vi "tm_getrange_a.vi"(8 "error in (no error)":errorcluster, 10 "Parameter":u32(ring)=4215968 items=["SENSOR MODE"=4212128, "CCD MODE"=4212384, "READOUT MODE"=4211872, "ACTIVE VIEW INDEX"=4343136, "BITS PER CHANNEL"=4342976, "IMAGE PIXEL TYPE"=4343296, "BINNING"=4215968, "EXPOSURE TIME"=2049184, "CONTRAST GAIN"=3163312, "CONTRAST OFFSET"=3163328, "LIGHT MODE"=2114720, "SENSITIVITY"=2114992, "PHOTON IMAGING MODE"=2115200, "HIGH DYNAMIC RANGE MODE"=3163360, "WHITE BALANCE"=3163568, "TEMPERATURE"=2115232, "TEMPERATURE TARGET"=2115264, "SENSOR COOLER FAN"=2115296, "LINEBUNDLE HEIGHT"=4212192, "MECHANICAL SHUTTER"=2115488, "BACK FOCUS POSITION"=8422304, "TRIGGER CONNECTOR"=1066432, "TRIGGER SOURCE"=1066144, "OUTPUT TRIGGER SOURCE"=1852576, "TRIGGER GLOBAL EXPOSURE"=2049680, "FIRST TRIGGER BEHAVIOR"=2049696, "CHANNEL SYNC"=1852352, "READOUT DIRECTION"=4211904, "PRE HSYNC COUNT"=1852704, "INTERNAL LINE SPEED"=4191408, "INTERNAL LINE INVERVAL"=4191424], 11 "Handle in":u32) -> (0 "error out":errorcluster, 1 "default":dbl, 2 "Range":cluster{"min":dbl, "max":dbl, "step":dbl}, 3 "Handle out":u32, 4 "Value Names":cluster{"Name":string, "Value":dbl}[](array[cluster]), 5 "Writable":bool, 6 "Text Values":bool)   [LabVIEW 2012]
uses:
  tmcamcon.dll
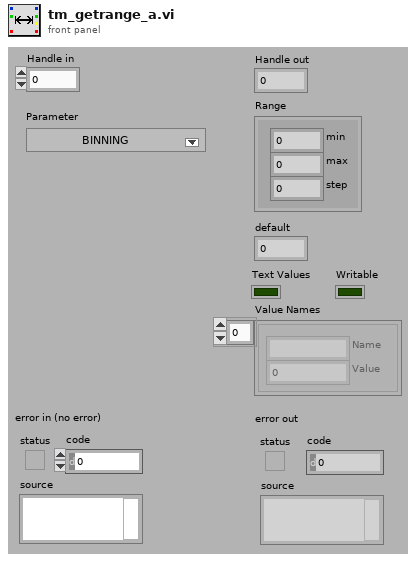
[diagram p1: front panel]
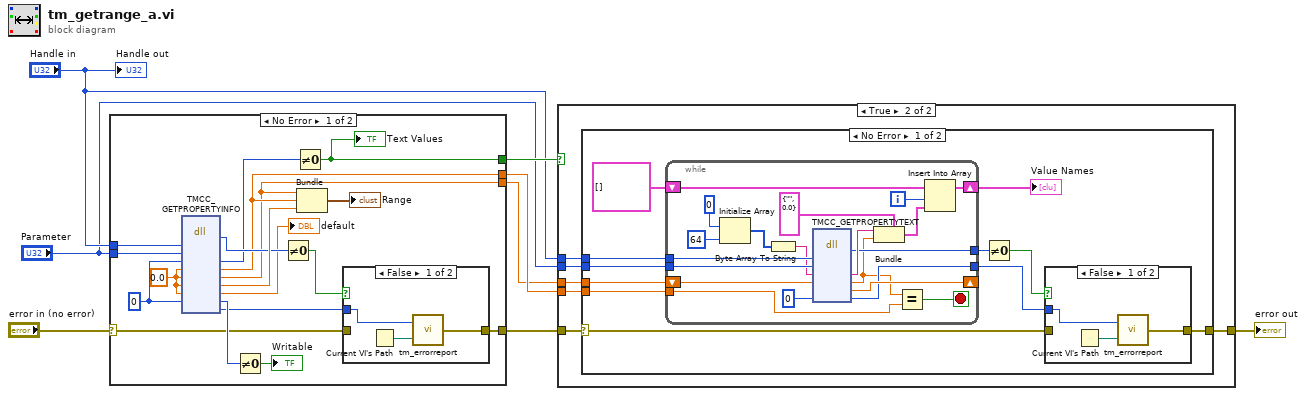
[diagram p0: block diagram]
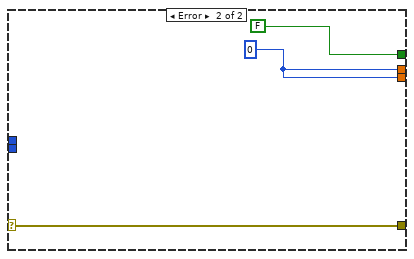
[diagram p6: hidden frame]
diagram:
  n1 = case shown="No Error" "error in (no error)" {
    selector: "error in (no error)" -> [w12 w33]
    tunnel: [w9 w33] -> w6
    tunnel: "Parameter" -> [w26 _]
    tunnel: "Handle in" -> [w20 _]
    tunnel: [w18 w31] -> w4
    tunnel: [w17 w31] -> w3
    tunnel: [w19 FALSE] -> w7
    frame No Error {
      w25 = 0.0
      w13 = u32 0
      n2 = dll-call lib="tmcamcon.dll" fn="TMCC_GETPROPERTYINFO"("HDCAM"=w20, "propertyid"=w26, "text"=w13, "max"=w25, "min"=w25, "step"=w25, "default"=w25, "writable"=w13) -> (w22:u32, "text"=w21:u32, "max"=w18:dbl, "min"=w17:dbl, "step"=w23:dbl, "default"=→"default":dbl, "writable"=w14:u32, "Erval"=w11:i32)  [unwired: 6 in, 2 out]
      n3 = Not Equal To 0?(x=w14) -> (x != 0?=→"Writable":bool)
      n4 = Not Equal To 0?(x=w22) -> (x != 0?=w10:bool)
      n5 = Not Equal To 0?(x=w21) -> (x != 0?=w19:bool)
      "Text Values" <- w19
      n6 = Bundle("min"=w17, "max"=w18, "step"=w23) -> (→"Range":cluster{"min":dbl, "max":dbl, "step":dbl})  [unwired: 1 in]
      n7 = case shown="False" w10 {
        tunnel: w12 -> [_ w30]
        tunnel: [w28 w30] -> w9
        tunnel: w11 -> [w27 _]
        frame False {
          n8 = Current VI's Path() -> (path=w29:path)
          n9 = call "tm_errorreport.vi"("Source"=w29, "Error"=w27) -> ("error out"=w28:errorcluster)
        }
        frame True {
        }
      }
    }
    frame Error {
      w31 = 0
    }
  }
  n10 = case shown="True" w7 {
    tunnel: w6 -> [w34 w40]
    tunnel: "Handle in" -> [_ w39]
    tunnel: "Parameter" -> [_ w38]
    tunnel: w3 -> [_ w37]
    tunnel: w4 -> [_ w36]
    tunnel: [w34 w35] -> w5
    frame False {
    }
    frame True {
      n11 = case shown="No Error" w40 {
        selector: w40 -> [w44 w76]
        tunnel: [w41 w76] -> w35
        tunnel: w39 -> [w48 _]
        tunnel: w38 -> [w47 _]
        tunnel: w37 -> [w46 _]
        tunnel: w36 -> [w45 _]
        frame No Error {
          n12 = while {
            shift-right: [w74] -> w50
            shift-left: cluster{"Name":string, "Value":dbl}[] [] ("Value Names") -> [w75]
            tunnel: [w71] -> w49
            tunnel: w48 -> [w69]
            tunnel: w47 -> [w68]
            shift-right: [w66] -> _
            shift-left: w46 -> [w67]
            tunnel: [w63] -> w43
            tunnel: w45 -> [w62]
            i -> [w70]
            stop <- w60 stop-if-true
            n13 = Initialize Array(u8 0, 64) -> (w57:u8[])
            n14 = Byte Array To String(unsigned byte array=w57) -> (string=w56:string)
            n15 = dll-call lib="tmcamcon.dll" fn="TMCC_GETPROPERTYTEXT"("HDCAM"=w69, "propertyid"=w68, "name"=w56, "value"=w67, "Erval"=0) -> (w71:u32, "name"=w72:string, "value"=w61:dbl, "nextvalue"=w66:dbl, "Erval"=w63:i32)  [unwired: 6 in, 2 out]
            n16 = Bundle(cluster=cluster{"name":string, "value":dbl} {"name"="", "value"=0.0}, "name"=w72, "value"=w61) -> (w73:cluster{"name":string, "value":dbl})
            n17 = Equal?(x=w61, y=w62) -> (x = y?=w60:bool)
            n18 = Insert Into Array(array=w75, index=w70, new element=w73) -> (w74:cluster{"Name":string, "Value":dbl}[])
          }
          "Value Names" <- w50
          n19 = Not Equal To 0?(x=w49) -> (x != 0?=w42:bool)
          n20 = case shown="False" w42 {
            tunnel: w44 -> [_ w55]
            tunnel: [w53 w55] -> w41
            tunnel: w43 -> [w52 _]
            frame False {
              n21 = Current VI's Path() -> (path=w54:path)
              n22 = call "tm_errorreport.vi"("Source"=w54, "Error"=w52) -> ("error out"=w53:errorcluster)
            }
            frame True {
            }
          }
        }
        frame Error {
        }
      }
    }
  }
  "error out" <- w5
  "Handle out" <- "Handle in"
